vi "PhysicalDAQmxChannels.vi"(8 "error in (no error)":errorcluster, 11 "Channel type":T1(ring)) -> (0 "error out":errorcluster, 3 "Channels of elected type":tag[](array[tag]))   [LabVIEW 2013]
uses:
  Program Files (x86)/National Instruments/LabVIEW 2013/user.lib/_OpenG.lib/array/array.llb/Conditional Auto-Indexing Tunnel (String)__ogtk.vi
  <resource>/objmgr/daqmx.rc
panel:
  out "transposed array":tag[][](array[tag])
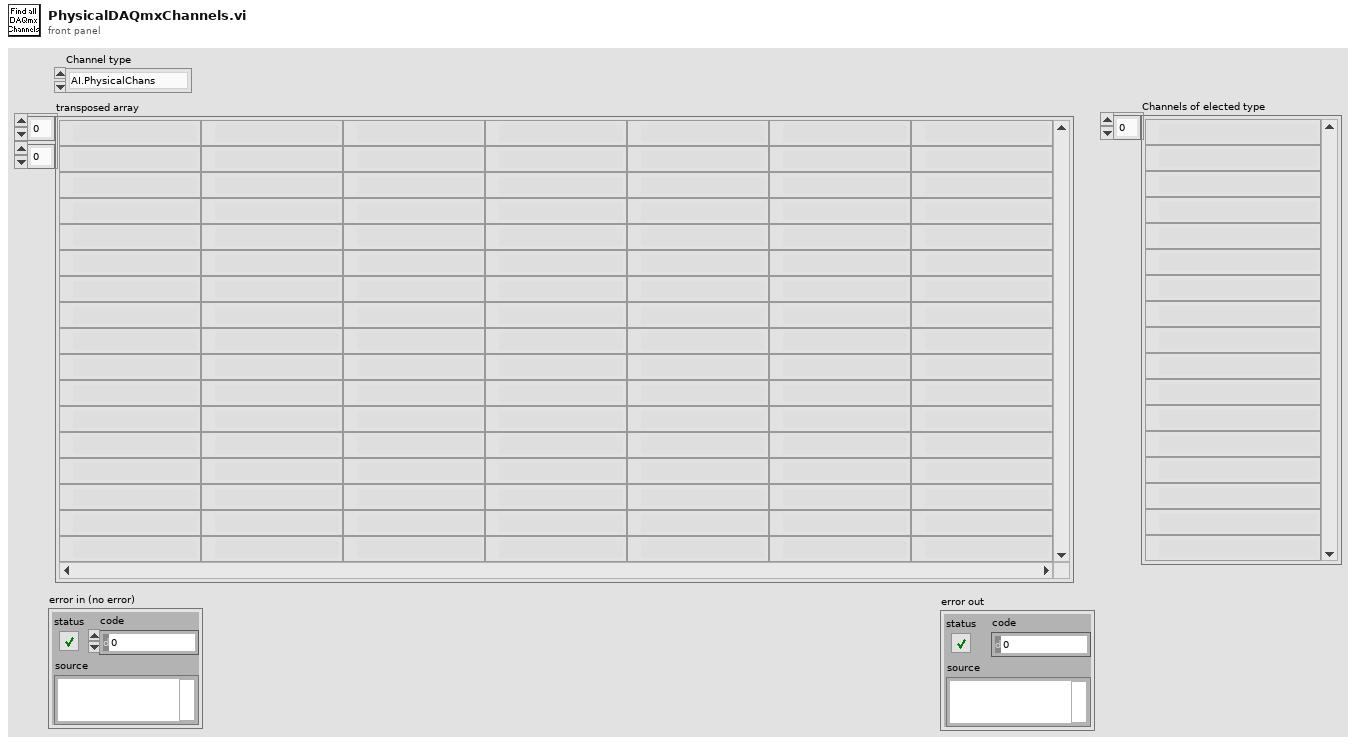
[diagram p1: front panel]
types:
  T1 = enum16{"AI.PhysicalChans", "AO.PhysicalChans", "DI.Ports", "DO.Ports", "CtrIn.PhysicalChans", "CtrOut.PhysicalChans"}
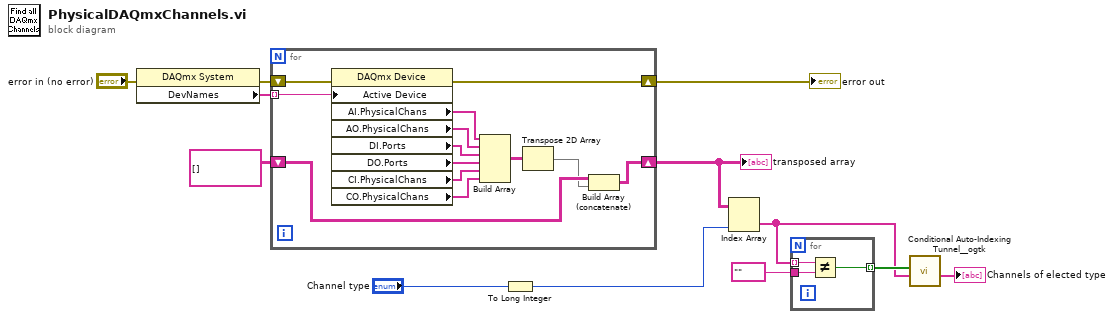
[diagram p0: block diagram]
diagram:
  n1 = property on="Property Node" class="DAQmx System"(error in="error in (no error)") -> (error out=w11:errorcluster, "DevNames"=w12:tag[])  [unwired: 1 in, 1 out]
  n2 = for {
    tunnel: w12 -> [w25] mode=indexing
    shift-right: [w15] -> w1
    shift-left: tag[][] [] -> [w14]
    shift-right: [w18] -> w10
    shift-left: w11 -> [w17]
    n3 = property class="DAQmx Device"(error in=w17, "Active Device"=w25) -> (error out=w18:errorcluster, "AI.PhysicalChans"=w24:tag[], "AO.PhysicalChans"=w23:tag[], "DI.Ports"=w22:tag[], "DO.Ports"=w21:tag[], "CI.PhysicalChans"=w20:tag[], "CO.PhysicalChans"=w19:tag[])  [unwired: 1 in, 1 out]
    n4 = Build Array(w24, w23, w22, w21, w20, w19) -> (w16:tag[][])
    n5 = Transpose 2D Array(2D array=w16) -> (transposed array=w13:tag[][])
    n6 = Build Array (concatenate)(w14, w13) -> (w15:tag[][])
  }
  "error out" <- w10
  "transposed array" <- w1
  n7 = To Long Integer(number="Channel type") -> (32bit integer=w6:i32)
  n8 = Index Array(array=w1, index (col)=w6) -> (element=w3:tag[])  [unwired: 1 in]
  n9 = for {
    tunnel: w3 -> [w28] mode=indexing
    tunnel: tag "" -> [w27]
    tunnel: [w26] -> w4 mode=indexing
    n10 = Not Equal?(x=w28, y=w27) -> (x != y?=w26:bool)
  }
  n11 = call-poly "Conditional Auto-Indexing Tunnel__ogtk.vi"("Array in"=w3, "Elements to keep"=w4) -> ("Filtered Array out"=→"Channels of elected type":string[])  [unwired: 5 in]
